vi "communicatejob.vi"(0 "sample port":refnum<visa-resource-name>[](array[refnum]), 1 "condition":bool[](array[boolean]), 2 "send command":string[](array[string])) -> (4 "error":errorcluster[](array[cluster]), 6 "receive data":string[](array[string]), 7 "receive command":string[](array[string]), 8 "receive result":bool[](array[boolean]))   [LabVIEW 2012]
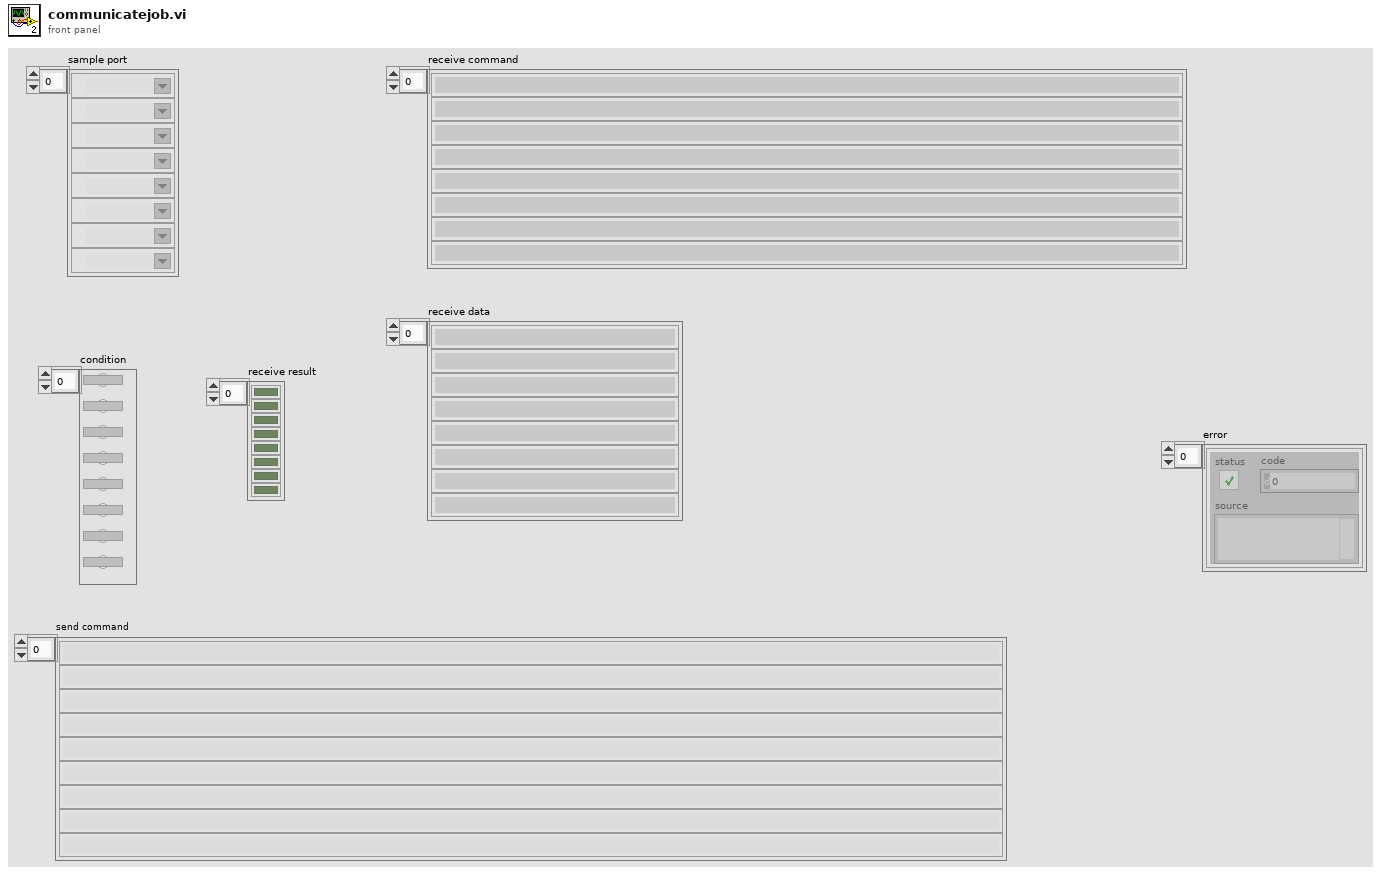
[diagram p1: front panel]
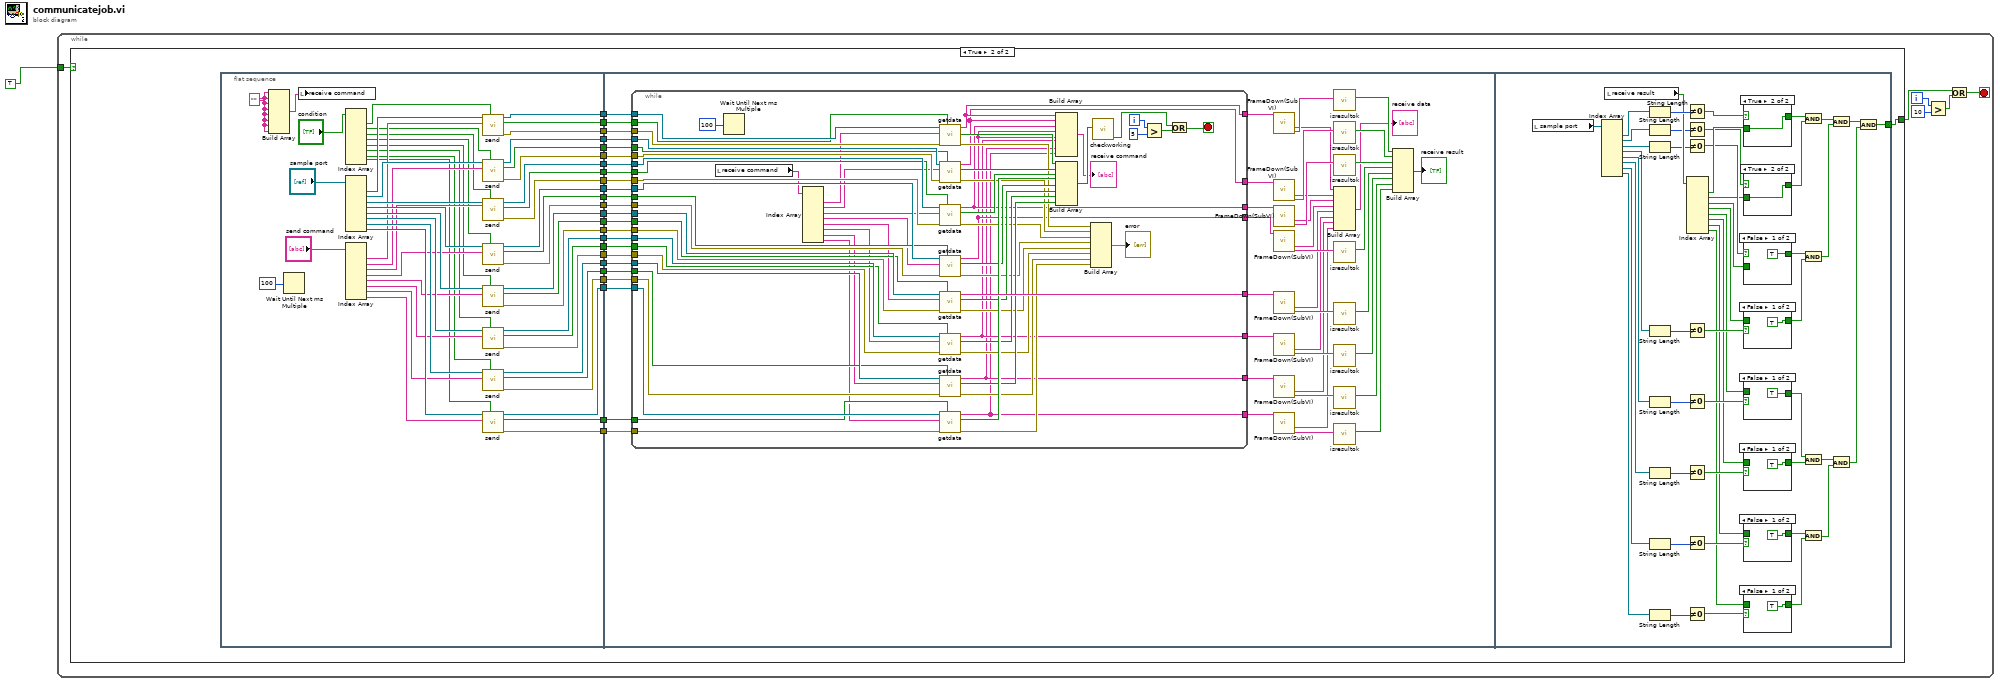
[diagram p0: block diagram]
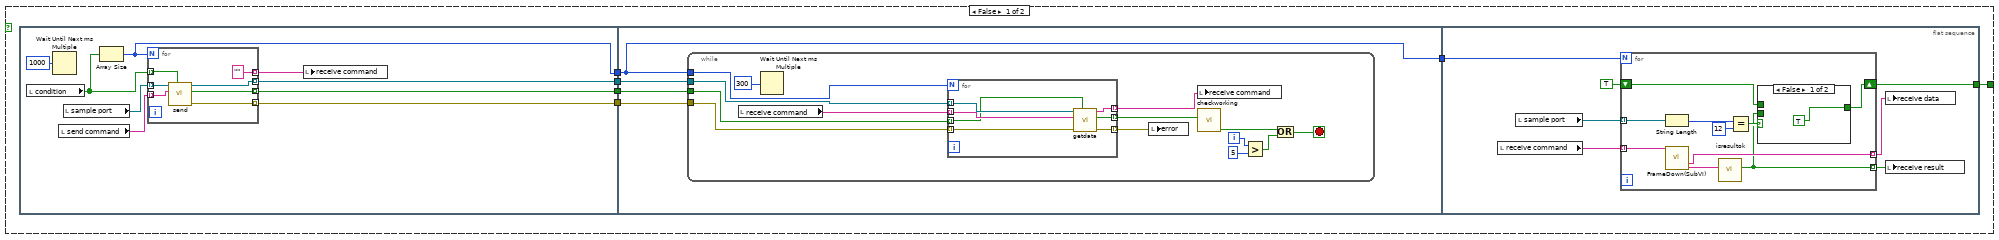
[diagram p2: hidden frame]
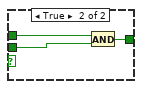
[diagram p3: hidden frame]
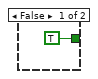
[diagram p10: hidden frame]
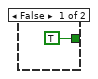
[diagram p11: hidden frame]
diagram:
  n1 = while {
    tunnel: TRUE -> [w2]
    i -> [w7]
    stop <- w5 stop-if-true
    n2 = case shown="True" w2 {
      tunnel: [w8 w76] -> w3
      frame False {
        n3 = flat-sequence {
          tunnel: [w18] -> w13
          tunnel: [w17] -> w12
          tunnel: [w16] -> w11
          tunnel: [w14] -> w10
          tunnel: w13 -> [w33]
          tunnel: w12 -> [w32]
          tunnel: w11 -> [w31]
          tunnel: w10 -> [w30]
          tunnel: [w30] -> w9
          tunnel: w9 -> [w61]
          tunnel: [w55] -> w8
          frame #0 {
            n4 = local read "condition"() -> (w20:bool[])
            n5 = Wait Until Next ms Multiple(millisecond multiple=1000) -> ()  [unwired: 1 out]
            n6 = local read "send command"() -> (w21:string[])
            n7 = local read "sample port"() -> (w22:refnum<visa-resource-name>[])
            n8 = Array Size(array=w20) -> (size(s)=w14:i32)
            n9 = for {
              N: w14 -> [_]
              tunnel: w22 -> [w29] mode=indexing
              tunnel: w21 -> [w28] mode=indexing
              tunnel: w20 -> [w27] mode=indexing
              tunnel: [""] -> w19 mode=indexing
              tunnel: [w25] -> w18 mode=indexing
              tunnel: [w24] -> w17 mode=indexing
              tunnel: [w23] -> w16 mode=indexing
              n10 = call "send.vi"("condition"=w27, "input"=w28, "port"=w29) -> ("error out"=w24:errorcluster, "condition"=w23:bool, "VISA resource name"=w25:refnum<visa-resource-name>)  [unwired: 6 in]
            }
            n11 = local write "receive command"(w19) -> ()
          }
          frame #1 {
            n12 = while {
              tunnel: w33 -> [w43]
              tunnel: w32 -> [w42]
              tunnel: w31 -> [w41]
              tunnel: w30 -> [w34]
              i -> [w39]
              stop <- w36 stop-if-true
              n13 = local read "receive command"() -> (w47:string[])
              n14 = Wait Until Next ms Multiple(millisecond multiple=300) -> ()  [unwired: 1 out]
              n15 = for {
                N: w34 -> [_]
                tunnel: w47 -> [w54] mode=indexing
                tunnel: [w53] -> w46 mode=indexing
                tunnel: [w52] -> w45 mode=indexing
                tunnel: [w51] -> w44 mode=indexing
                tunnel: w43 -> [w50] mode=indexing
                tunnel: w42 -> [w49] mode=indexing
                tunnel: w41 -> [w48] mode=indexing
                n16 = call "getdata.vi"("condition"=w48, "error in (no error)"=w49, "inputdata"=w54, "port"=w50) -> ("error out"=w51:errorcluster, "end"=w52:bool, "outputdata"=w53:string)  [unwired: 4 in, 1 out]
              }
              n17 = local write "error"(w44) -> ()
              n18 = local write "receive command"(w46) -> ()
              n19 = call "checkworking.vi"("Array"=w45) -> ("Boolean"=w37:bool)  [unwired: 8 in]
              n20 = Greater?(x=w39, y=5) -> (0:w38:bool)
              n21 = Or(x=w37, y=w38) -> (x .or. y?=w36:bool)
            }
          }
          frame #2 {
            n22 = local read "receive command"() -> (w60:string[])
            n23 = local read "sample port"() -> (w57:refnum<visa-resource-name>[])
            n24 = for {
              N: w61 -> [_]
              tunnel: w60 -> [w71] mode=indexing
              tunnel: [w69] -> w59 mode=indexing
              tunnel: [w64] -> w58 mode=indexing
              tunnel: w57 -> [w66] mode=indexing
              shift-right: [w63] -> w55
              shift-left: TRUE -> [w62]
              n25 = String Length(string=w66) -> (length=w67:i32)
              n26 = call "FrameDown(SubVI).vi"("input frame"=w71) -> ("data"=w69:string, "result"=w70:string)  [unwired: 4 in, 9 out]
              n27 = call "isresultok.vi"("result"=w70) -> ("ok"=w64:bool)  [unwired: 10 in]
              n28 = Equal?(x=w67, y=12) -> (x = y?=w65:bool)
              n29 = case shown="False" w65 {
                tunnel: w64 -> [_ w75]
                tunnel: [TRUE w74] -> w63
                tunnel: w62 -> [_ w73]
                frame False {
                }
                frame True {
                  n30 = And(x=w73, y=w75) -> (x .and. y?=w74:bool)
                }
              }
            }
            n31 = local write "receive data"(w59) -> ()
            n32 = local write "receive result"(w58) -> ()
          }
        }
      }
      frame True {
        n33 = flat-sequence {
          tunnel: [w127] -> w100
          tunnel: [w126] -> w99
          tunnel: [w125] -> w98
          tunnel: [w124] -> w97
          tunnel: [w123] -> w96
          tunnel: [w122] -> w95
          tunnel: [w121] -> w94
          tunnel: [w120] -> w93
          tunnel: [w119] -> w92
          tunnel: [w118] -> w91
          tunnel: [w117] -> w90
          tunnel: [w116] -> w89
          tunnel: [w115] -> w88
          tunnel: [w114] -> w87
          tunnel: [w113] -> w86
          tunnel: [w112] -> w85
          tunnel: [w111] -> w84
          tunnel: [w110] -> w83
          tunnel: [w109] -> w82
          tunnel: [w108] -> w81
          tunnel: [w107] -> w80
          tunnel: [w106] -> w79
          tunnel: [w105] -> w78
          tunnel: [w104] -> w77
          tunnel: w100 -> [w178]
          tunnel: w99 -> [w177]
          tunnel: w98 -> [w176]
          tunnel: w97 -> [w175]
          tunnel: w96 -> [w174]
          tunnel: w95 -> [w173]
          tunnel: w94 -> [w172]
          tunnel: w93 -> [w171]
          tunnel: w92 -> [w170]
          tunnel: w91 -> [w169]
          tunnel: w90 -> [w168]
          tunnel: w89 -> [w167]
          tunnel: w88 -> [w166]
          tunnel: w87 -> [w165]
          tunnel: w86 -> [w164]
          tunnel: w85 -> [w163]
          tunnel: w84 -> [w162]
          tunnel: w83 -> [w161]
          tunnel: w82 -> [w160]
          tunnel: w81 -> [w159]
          tunnel: w80 -> [w158]
          tunnel: w79 -> [w157]
          tunnel: w78 -> [w156]
          tunnel: w77 -> [w155]
          tunnel: [w279] -> w76
          frame #0 {
            w102 = ""
            n34 = Build Array(w102, w102, w102, w102, w102, w102, w102, w102) -> (w103:string[])
            n35 = Wait Until Next ms Multiple(millisecond multiple=100) -> ()  [unwired: 1 out]
            n36 = local write "receive command"(w103) -> ()
            n37 = Index Array(array="condition") -> (element #1=w135:bool, element #2=w134:bool, element #3=w133:bool, element #4=w132:bool, element #5=w131:bool, element #6=w130:bool, element #7=w129:bool, element #8=w128:bool)  [unwired: 8 in]
            n38 = Index Array(array="sample port") -> (element #1=w153:refnum<visa-resource-name>, element #2=w152:refnum<visa-resource-name>, element #3=w151:refnum<visa-resource-name>, element #4=w150:refnum<visa-resource-name>, element #5=w149:refnum<visa-resource-name>, element #6=w148:refnum<visa-resource-name>, element #7=w147:refnum<visa-resource-name>, element #8=w146:refnum<visa-resource-name>)  [unwired: 8 in]
            n39 = Index Array(array="send command") -> (element #1=w145:string, element #2=w144:string, element #3=w143:string, element #4=w142:string, element #5=w141:string, element #6=w140:string, element #7=w139:string, element #8=w138:string)  [unwired: 8 in]
            n40 = call "send.vi"("condition"=w135, "input"=w145, "port"=w153) -> ("error out"=w126:errorcluster, "condition"=w111:bool, "VISA resource name"=w127:refnum<visa-resource-name>)  [unwired: 6 in]
            n41 = call "send.vi"("condition"=w134, "input"=w144, "port"=w152) -> ("error out"=w124:errorcluster, "condition"=w110:bool, "VISA resource name"=w125:refnum<visa-resource-name>)  [unwired: 6 in]
            n42 = call "send.vi"("condition"=w133, "input"=w143, "port"=w151) -> ("error out"=w122:errorcluster, "condition"=w109:bool, "VISA resource name"=w123:refnum<visa-resource-name>)  [unwired: 6 in]
            n43 = call "send.vi"("condition"=w132, "input"=w142, "port"=w150) -> ("error out"=w120:errorcluster, "condition"=w108:bool, "VISA resource name"=w121:refnum<visa-resource-name>)  [unwired: 6 in]
            n44 = call "send.vi"("condition"=w131, "input"=w141, "port"=w149) -> ("error out"=w118:errorcluster, "condition"=w104:bool, "VISA resource name"=w119:refnum<visa-resource-name>)  [unwired: 6 in]
            n45 = call "send.vi"("condition"=w130, "input"=w140, "port"=w148) -> ("error out"=w116:errorcluster, "condition"=w105:bool, "VISA resource name"=w117:refnum<visa-resource-name>)  [unwired: 6 in]
            n46 = call "send.vi"("condition"=w129, "input"=w139, "port"=w147) -> ("error out"=w114:errorcluster, "condition"=w106:bool, "VISA resource name"=w115:refnum<visa-resource-name>)  [unwired: 6 in]
            n47 = call "send.vi"("condition"=w128, "input"=w138, "port"=w146) -> ("error out"=w112:errorcluster, "condition"=w107:bool, "VISA resource name"=w113:refnum<visa-resource-name>)  [unwired: 6 in]
          }
          frame #1 {
            n48 = while {
              tunnel: w178 -> [w262]
              tunnel: w177 -> [w261]
              tunnel: w176 -> [w260]
              tunnel: w175 -> [w259]
              tunnel: w174 -> [w258]
              tunnel: w173 -> [w257]
              tunnel: w172 -> [w256]
              tunnel: w171 -> [w255]
              tunnel: w170 -> [w254]
              tunnel: w169 -> [w253]
              tunnel: w168 -> [w252]
              tunnel: w167 -> [w251]
              tunnel: w166 -> [w250]
              tunnel: w165 -> [w249]
              tunnel: w164 -> [w248]
              tunnel: w163 -> [w247]
              tunnel: w162 -> [w237]
              tunnel: w161 -> [w236]
              tunnel: w160 -> [w235]
              tunnel: w159 -> [w234]
              tunnel: w158 -> [w233]
              tunnel: w157 -> [w232]
              tunnel: w156 -> [w231]
              tunnel: w155 -> [w230]
              tunnel: [w229] -> w197
              tunnel: [w228] -> w196
              tunnel: [w227] -> w195
              tunnel: [w226] -> w194
              tunnel: [w225] -> w192
              tunnel: [w278] -> w193
              tunnel: [w224] -> w191
              tunnel: [w223] -> w190
              i -> [w266]
              stop <- w263 stop-if-true
              n49 = local read "receive command"() -> (w221:string[])
              n50 = Wait Until Next ms Multiple(millisecond multiple=100) -> ()  [unwired: 1 out]
              n51 = Index Array(array=w221) -> (element #1=w220:string, element #2=w219:string, element #3=w218:string, element #4=w217:string, element #5=w216:string, element #6=w215:string, element #7=w214:string, element #8=w213:string)  [unwired: 8 in]
              n52 = call "getdata.vi"("condition"=w237, "error in (no error)"=w261, "inputdata"=w220, "port"=w262) -> ("error out"=w239:errorcluster, "end"=w277:bool, "outputdata"=w229:string)  [unwired: 4 in, 1 out]
              n53 = call "getdata.vi"("condition"=w236, "error in (no error)"=w259, "inputdata"=w219, "port"=w260) -> ("error out"=w240:errorcluster, "end"=w276:bool, "outputdata"=w228:string)  [unwired: 4 in, 1 out]
              n54 = call "getdata.vi"("condition"=w235, "error in (no error)"=w257, "inputdata"=w218, "port"=w258) -> ("error out"=w241:errorcluster, "end"=w275:bool, "outputdata"=w227:string)  [unwired: 4 in, 1 out]
              n55 = call "getdata.vi"("condition"=w234, "error in (no error)"=w255, "inputdata"=w217, "port"=w256) -> ("error out"=w242:errorcluster, "end"=w273:bool, "outputdata"=w226:string)  [unwired: 4 in, 1 out]
              n56 = call "getdata.vi"("condition"=w230, "error in (no error)"=w253, "inputdata"=w216, "port"=w254) -> ("error out"=w243:errorcluster, "end"=w272:bool, "outputdata"=w278:string)  [unwired: 4 in, 1 out]
              n57 = call "getdata.vi"("condition"=w231, "error in (no error)"=w251, "inputdata"=w215, "port"=w252) -> ("error out"=w244:errorcluster, "end"=w271:bool, "outputdata"=w225:string)  [unwired: 4 in, 1 out]
              n58 = call "getdata.vi"("condition"=w232, "error in (no error)"=w249, "inputdata"=w214, "port"=w250) -> ("error out"=w245:errorcluster, "end"=w270:bool, "outputdata"=w224:string)  [unwired: 4 in, 1 out]
              n59 = call "getdata.vi"("condition"=w233, "error in (no error)"=w247, "inputdata"=w213, "port"=w248) -> ("error out"=w246:errorcluster, "end"=w274:bool, "outputdata"=w223:string)  [unwired: 4 in, 1 out]
              n60 = Build Array(w229, w228, w227, w226, w226, w225, w224, w223) -> (→"receive command":string[])
              n61 = Build Array(w277, w276, w275, w274, w273, w272, w271, w270) -> (w269:bool[])
              n62 = Build Array(w239, w240, w241, w242, w243, w244, w245, w246) -> (→"error":errorcluster[])
              n63 = call "checkworking.vi"("Array"=w269) -> ("Boolean"=w265:bool)  [unwired: 8 in]
              n64 = Greater?(x=w266, y=5) -> (0:w264:bool)
              n65 = Or(x=w265, y=w264) -> (x .or. y?=w263:bool)
            }
            n66 = call "FrameDown(SubVI).vi"("input frame"=w197) -> ("data"=w187:string, "result"=w211:string)  [unwired: 4 in, 9 out]
            n67 = call "FrameDown(SubVI).vi"("input frame"=w196) -> ("data"=w186:string, "result"=w206:string)  [unwired: 4 in, 9 out]
            n68 = call "FrameDown(SubVI).vi"("input frame"=w195) -> ("data"=w185:string, "result"=w209:string)  [unwired: 4 in, 9 out]
            n69 = call "FrameDown(SubVI).vi"("input frame"=w194) -> ("data"=w184:string, "result"=w212:string)  [unwired: 4 in, 9 out]
            n70 = call "FrameDown(SubVI).vi"("input frame"=w193) -> ("data"=w183:string, "result"=w207:string)  [unwired: 4 in, 9 out]
            n71 = call "FrameDown(SubVI).vi"("input frame"=w192) -> ("data"=w182:string, "result"=w210:string)  [unwired: 4 in, 9 out]
            n72 = call "FrameDown(SubVI).vi"("input frame"=w191) -> ("data"=w181:string, "result"=w208:string)  [unwired: 4 in, 9 out]
            n73 = call "FrameDown(SubVI).vi"("input frame"=w190) -> ("data"=w180:string, "result"=w189:string)  [unwired: 4 in, 9 out]
            n74 = call "isresultok.vi"("result"=w211) -> ("ok"=w205:bool)  [unwired: 10 in]
            n75 = call "isresultok.vi"("result"=w206) -> ("ok"=w204:bool)  [unwired: 10 in]
            n76 = call "isresultok.vi"("result"=w209) -> ("ok"=w203:bool)  [unwired: 10 in]
            n77 = Build Array(w187, w186, w185, w184, w183, w182, w181, w180) -> (→"receive data":string[])
            n78 = call "isresultok.vi"("result"=w212) -> ("ok"=w202:bool)  [unwired: 10 in]
            n79 = call "isresultok.vi"("result"=w207) -> ("ok"=w201:bool)  [unwired: 10 in]
            n80 = call "isresultok.vi"("result"=w210) -> ("ok"=w200:bool)  [unwired: 10 in]
            n81 = call "isresultok.vi"("result"=w208) -> ("ok"=w199:bool)  [unwired: 10 in]
            n82 = call "isresultok.vi"("result"=w189) -> ("ok"=w188:bool)  [unwired: 10 in]
            n83 = Build Array(w205, w204, w203, w202, w201, w200, w199, w188) -> (→"receive result":bool[])
          }
          frame #2 {
            n84 = local read "sample port"() -> (w327:refnum<visa-resource-name>[])
            n85 = Index Array(array=w327) -> (element #1=w326:refnum<visa-resource-name>, element #2=w316:refnum<visa-resource-name>, element #3=w315:refnum<visa-resource-name>, element #4=w308:refnum<visa-resource-name>, element #5=w307:refnum<visa-resource-name>, element #6=w296:refnum<visa-resource-name>, element #7=w289:refnum<visa-resource-name>, element #8=w288:refnum<visa-resource-name>)  [unwired: 8 in]
            n86 = local read "receive result"() -> (w322:bool[])
            n87 = String Length(string=w326) -> (length=w325:i32)
            n88 = String Length(string=w316) -> (length=w320:i32)
            n89 = String Length(string=w315) -> (length=w318:i32)
            n90 = String Length(string=w308) -> (length=w312:i32)
            n91 = String Length(string=w307) -> (length=w310:i32)
            n92 = String Length(string=w296) -> (length=w300:i32)
            n93 = String Length(string=w289) -> (length=w295:i32)
            n94 = String Length(string=w288) -> (length=w292:i32)
            n95 = Not Equal To 0?(x=w325) -> (x != 0?=w324:bool)
            n96 = Not Equal To 0?(x=w320) -> (x != 0?=w319:bool)
            n97 = Not Equal To 0?(x=w318) -> (x != 0?=w317:bool)
            n98 = Not Equal To 0?(x=w312) -> (x != 0?=w311:bool)
            n99 = Not Equal To 0?(x=w310) -> (x != 0?=w309:bool)
            n100 = Not Equal To 0?(x=w300) -> (x != 0?=w299:bool)
            n101 = Not Equal To 0?(x=w295) -> (x != 0?=w294:bool)
            n102 = Not Equal To 0?(x=w292) -> (x != 0?=w291:bool)
            n103 = Index Array(array=w322) -> (element #1=w321:bool, element #2=w313:bool, element #3=w304:bool, element #4=w303:bool, element #5=w302:bool, element #6=w297:bool, element #7=w287:bool, element #8=w286:bool)  [unwired: 8 in]
            n104 = case shown="True" w324 {
              tunnel: w321 -> [_ w343]
              tunnel: [TRUE w343] -> w323
              frame False {
              }
              frame True {
              }
            }
            n105 = case shown="True" w319 {
              tunnel: w313 -> [_ w341]
              tunnel: [TRUE w341] -> w314
              frame False {
              }
              frame True {
              }
            }
            n106 = case shown="False" w317 {
              tunnel: [TRUE w339] -> w305
              tunnel: w304 -> [_ w339]
              frame False {
              }
              frame True {
              }
            }
            n107 = case shown="False" w311 {
              tunnel: [TRUE w337] -> w306
              tunnel: w303 -> [_ w337]
              frame False {
              }
              frame True {
              }
            }
            n108 = case shown="False" w309 {
              tunnel: [TRUE w335] -> w301
              tunnel: w302 -> [_ w335]
              frame False {
              }
              frame True {
              }
            }
            n109 = case shown="False" w299 {
              tunnel: [TRUE w333] -> w298
              tunnel: w297 -> [_ w333]
              frame False {
              }
              frame True {
              }
            }
            n110 = case shown="False" w294 {
              tunnel: [TRUE w331] -> w293
              tunnel: w287 -> [_ w331]
              frame False {
              }
              frame True {
              }
            }
            n111 = case shown="False" w291 {
              tunnel: [TRUE w329] -> w290
              tunnel: w286 -> [_ w329]
              frame False {
              }
              frame True {
              }
            }
            n112 = And(x=w323, y=w314) -> (x .and. y?=w285:bool)
            n113 = And(x=w305, y=w306) -> (x .and. y?=w284:bool)
            n114 = And(x=w301, y=w298) -> (x .and. y?=w283:bool)
            n115 = And(x=w293, y=w290) -> (x .and. y?=w282:bool)
            n116 = And(x=w285, y=w284) -> (x .and. y?=w280:bool)
            n117 = And(x=w283, y=w282) -> (x .and. y?=w281:bool)
            n118 = And(x=w280, y=w281) -> (x .and. y?=w279:bool)
          }
        }
      }
    }
    n119 = Greater?(x=w7, y=u16 10) -> (0:w4:bool)
    n120 = Or(x=w3, y=w4) -> (x .or. y?=w5:bool)
  }
